vi "Start Arduino Comms.vi"(1 "Arduino comm. params.":T1={"VISA resource name"="COM9", "byte count"=64, "flow control (0:none)"=0, "stop bits (10: 1 bit)"=10, "parity (0:none)"=enum."None", "data bits (8)"=8, "termination char "=10, "Enable Termination\nChar"=TRUE, "baud rate (bps)"=115200, "timeout (ms)"=1000, "Locked"=FALSE} {"termination char" format="%02x"; "data bits (8)" min=5 max=8 step=1; "stop bits (10: 1 bit)" items=["1.0"=10, "1.5"=15, "2.0"=20]; "flow control (0:none)" items=["None", "XON/XOFF", "RTS/CTS", "XON/XOFF & RTS/CTS", "DTR/DSR", "XON/XOFF & DTR/DSR"]}) -> (0 "Error":errorcluster)   [LabVIEW 2012]
uses:
  Arduino_comm_params.ctl
  Arduino_comms_Global.vi
  <vilib>/Instr/_visa.llb/VISA Configure Serial Port (Instr).vi
panel:
  # "(0xA = '\\n' = newline)"
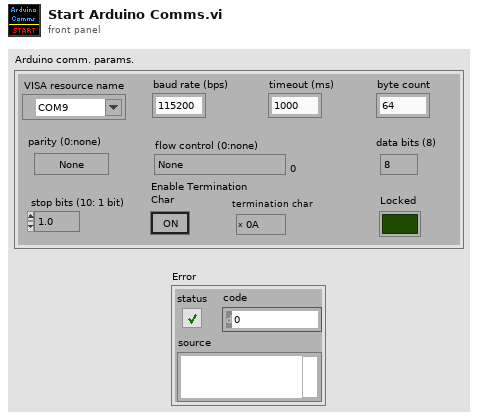
[diagram p1: front panel]
types:
  T1 = typedef "Arduino_comm_params.ctl" = cluster{"VISA resource name":refnum<visa-resource-name>, "byte count":u32, "flow control (0:none)":u16, "stop bits (10: 1 bit)":u16, "parity (0:none)":enum16{"None", "Odd", "Even", "Mark", "Space"}, "data bits (8)":u16, "termination char ":u8, "Enable Termination\nChar":bool, "baud rate (bps)":u32, "timeout (ms)":u32, "Locked":bool}
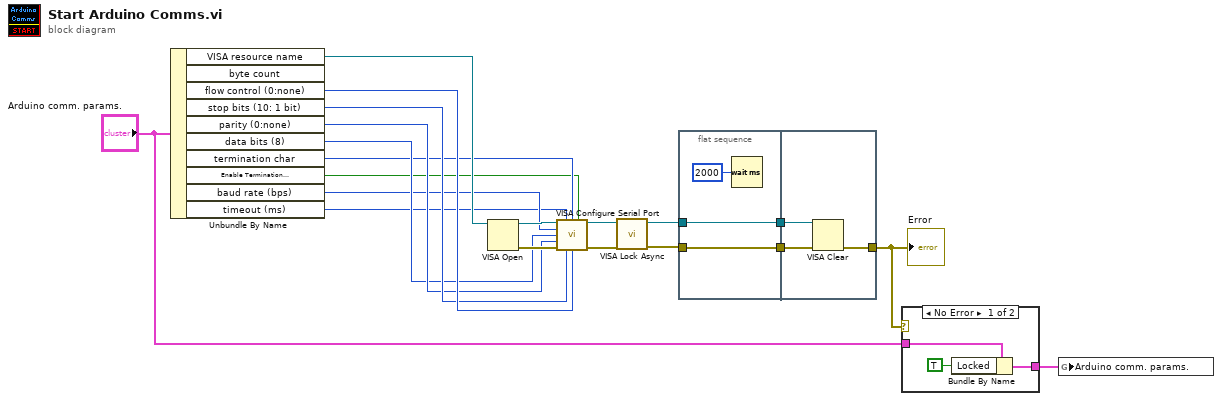
[diagram p0: block diagram]
diagram:
  n1 = Unbundle By Name("Arduino comm. params.") -> ("VISA resource name"=w13:refnum<visa-resource-name>, "flow control (0:none)"=w12:u16, "stop bits (10: 1 bit)"=w11:u16, "parity (0:none)"=w10:enum16{"None", "Odd", "Even", "Mark", "Space"}, "data bits (8)"=w9:u16, "termination char"=w6:u8, "Enable Termination\nChar"=w5:bool, "baud rate (bps)"=w8:u32, "timeout (ms)"=w7:u32)  [unwired: 1 out]
  n2 = VISA Open(VISA resource name=w13) -> (VISA resource name=w18:refnum<visa-resource-name>, error out=w17:errorcluster)  [unwired: 4 in]
  n3 = call-poly "VISA Configure Serial Port"("VISA resource name"=w18, "timeout (10sec)"=w7, "termination char\n(0xA = '\\n' = LF)"=w6, "Enable Termination\nChar (T)"=w5, "baud rate (9600)"=w8, "data bits (8)"=w9, "parity (0:none)"=w10, "error in (no error)"=w17, "stop bits (10: 1 bit)"=w11, "flow control (0:none)"=w12) -> ("VISA resource name out"=w16:refnum<visa-resource-name>, "error out"=w15:errorcluster)  [unwired: 4 in]
  n4 = call <vilib>:"VISA Lock Async.vi"("error in (no error)"=w15, "VISA resource name"=w16) -> ("error out"=w14:errorcluster, "VISA resource name out"=w4:refnum<visa-resource-name>)  [unwired: 7 in, 1 out]
  n5 = flat-sequence {
    tunnel: w14 -> [w22]
    tunnel: w4 -> [w23]
    tunnel: [w23] -> w20
    tunnel: [w22] -> w19
    tunnel: w19 -> [w25]
    tunnel: w20 -> [w26]
    tunnel: [w24] -> w2
    frame #0 {
      n6 = Wait (ms)(milliseconds to wait=u32 2000) -> ()  [unwired: 1 out]
    }
    frame #1 {
      n7 = VISA Clear(VISA resource name=w26, error in (no error)=w25) -> (error out=w24:errorcluster)  [unwired: 1 out]
    }
  }
  n8 = case shown="No Error" w2 {
    tunnel: [w27 w30] -> w3
    tunnel: "Arduino comm. params." -> [w28 w30]
    frame No Error {
      n9 = Bundle By Name(cluster=w28, "Locked"=TRUE) -> (w27:T1)
    }
    frame Error {
    }
  }
  n10 = global write "Arduino_comms_Global.vi" "Arduino comm. params."(w3) -> ()
  "Error" <- w2
